vi "init.vi"() -> ()   [LabVIEW 2015]
uses:
  <vilib>/LabVIEW Interface for Arduino/Type Defs/Pin Mode.ctl
  <vilib>/LabVIEW Interface for Arduino/Type Defs/Board Type.ctl
  <vilib>/LabVIEW Interface for Arduino/Type Defs/Connection Type.ctl
  <vilib>/LabVIEW Interface for Arduino/LabVIEW Interface for Arduino.lvlib
panel:
  in  "stop":bool
  in  "LED":bool
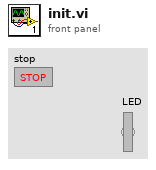
[diagram p1: front panel]
types:
  T1 = typedef "LabVIEW Interface for Arduino.lvlib/Connection Type.ctl" = enum8{"USB / Serial", "XBEE", "BlueSmirf (Bluetooth)"}
  T2 = typedef "LabVIEW Interface for Arduino.lvlib/Board Type.ctl" = enum16{"Uno", "Dimuelanove w/Atmega 328", "Mega 2560"}
  T3 = typedef "LabVIEW Interface for Arduino.lvlib/Pin Mode.ctl" = enum8{"Input", "Output"}
  T4 = typedef "LabVIEW Interface for Arduino.lvlib/Arduino Resource.ctl" = cluster{"VISA resource":refnum<visa-resource-name>, "Board Type":T2, "Connection Type":enum8{"USB / Serial"}, "Bytes Per Packet (15)":u8}
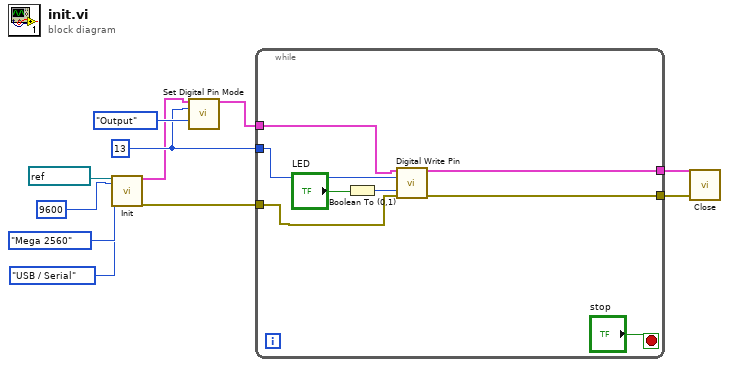
[diagram p0: block diagram]
diagram:
  w10 = u8 13 ("Digital I/O Pin")
  n1 = call <vilib>:"Init.vi"("VISA resource"=refnum<visa-resource-name> "COM7", "Baud Rate (115200)"=u32 9600, "Board Type (Uno)"=Board_Type."Mega 2560", "Connection Type (USB/Serial)"=Connection_Type."USB / Serial") -> ("Arduino Resource"=w8:T4, "error out"=w3:errorcluster)  [unwired: 14 in]
  n2 = call <vilib>:"Set Digital Pin Mode.vi"("Arduino Resource"=w8, "Digital I/O Pin"=w10, "Pin Mode (Input)"=Pin_Mode."Output") -> ("Arduino Resource"=w7:T4)  [unwired: 11 in, 1 out]
  n3 = while {
    tunnel: w10 -> [w18]
    tunnel: w7 -> [w19]
    tunnel: w3 -> [w16]
    tunnel: [w15] -> w2
    tunnel: [w14] -> w1
    stop <- "stop" stop-if-true
    n4 = Boolean To (0,1)(Boolean="LED") -> (0, 1=w17:i16)
    n5 = call <vilib>:"Digital Write Pin.vi"("Arduino Resource"=w19, "Digital I/O Pin (0)"=w18, "Value (0)"=w17, "error in"=w16) -> ("Arduino Resource"=w15:T4, "error out"=w14:errorcluster)  [unwired: 10 in]
  }
  n6 = call <vilib>:"Close.vi"("Arduino Resource"=w2, "error in"=w1) -> ()  [unwired: 13 in, 1 out]
